vi "_글로벌.vi"() -> ()   [LabVIEW 2014]
panel:
  in  "ROI":T1
  out "컬러1번 앞":dbl
  out "컬러2번":dbl
  out "컬러0번":dbl
  out "컬러1번 오":dbl
  out "2: 굴릴각도":dbl=60.0
  out "2: 공각도":dbl=233.0
  in  "Red or Hue 5":cluster{i32, i32}(slide)={0, 255} scale=0.0..255.0
  in  "Green or Saturation 5":cluster{i32, i32}(slide)={0, 30} scale=0.0..255.0
  in  "Blue or Luminance 5":cluster{i32, i32}(slide)={0, 55} scale=0.0..255.0
  in  "탭 컨트롤":enum32{"볼링핀 0", "녹색핀 1"}(tab)
  in  "Blue or Luminance":cluster{i32, i32}(slide)={135, 255} scale=0.0..255.0
  in  "Green or Saturation":cluster{i32, i32}(slide)={0, 55} scale=0.0..255.0
  in  "Red or Hue":cluster{i32, i32}(slide)={0, 255} scale=0.0..255.0
  in  "Blue or Luminance 3":cluster{i32, i32}(slide)={60, 255} scale=0.0..255.0
  in  "Green or Saturation 3":cluster{i32, i32}(slide)={35, 255} scale=0.0..255.0
  in  "Red or Hue 3":cluster{i32, i32}(slide)={50, 130} scale=0.0..255.0
  out "흰/검 반 값":dbl=0.15
  out "흰색과 밖 차이값":dbl=0.15
  out "6: 앞쪽각도":dbl=128.0
  out "6: 왼쪽각도":dbl=250.0
  out "5: 앞쪽각도":dbl=240.0
  out "5: 오른각도":dbl=120.0
  out "4: 뒷쪽각도":dbl
  out "4: 오른각도":dbl=122.0
  out "정지할 차이값":dbl=0.05
  # "배경색(검은색) 색조"
  # "255"
  # "채도"
  # "35"
  # "광도"
  # "60"
  # "흰색 : 0/255"
  # "흰색 : 0~55"
  # "흰색 : 135~255"
  # "녹색 : 50/130"
  # "녹색 : 35/255"
  # "녹색 : 60/255"
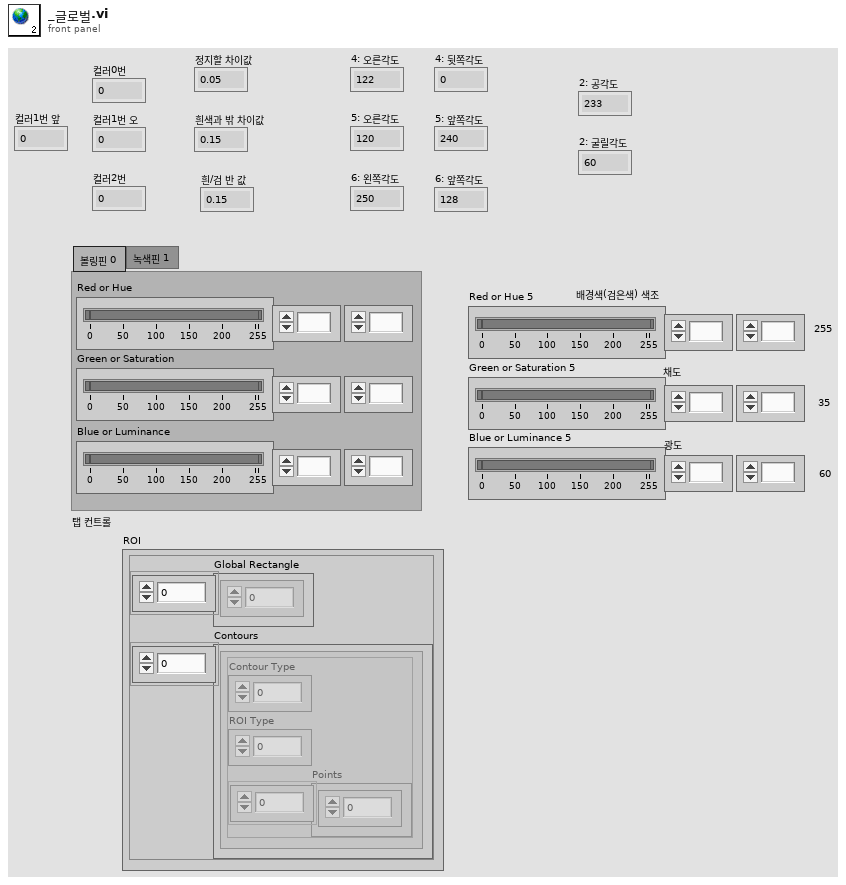
[diagram p1: front panel]
types:
  T1 = cluster{"Global Rectangle":i32[], "Contours":cluster{"Contour Type":u32, "ROI Type":u32, "Points":i32[]}[]}
diagram:
